vi "FSK_ROBOTIC_ARM_QR_FOUND.vi"() -> ()   [LabVIEW 2025]
uses:
  <vilib>/userDefined/High Color/IMAQdx.ctl
  Program Files/National Instruments/LabVIEW 2025/examples/Instrument IO/Serial/support/Serial - Settings.ctl
  Program Files/National Instruments/LabVIEW 2025/examples/Instrument IO/Serial/support/Serial - XON-XOFF Characters.ctl
  Program Files/National Instruments/LabVIEW 2025/examples/Instrument IO/Serial/support/Serial - ASCII Characters.ctl
  <vilib>/Instr/_visa.llb/VISA Configure Serial Port (Instr).vi
  <vilib>/vision/driver/NI_Vision_Acquisition_Software.lvlib
  <vilib>/vision/NI_Vision_Development_Module.lvlib
panel:
  in  "stop 2":bool
  in  "Termination Character":u8=10 format="%.0x"
  in  "End Write on Termination Character?":bool=TRUE
  in  "VISA resource name":refnum<visa-resource-name>="COM1"
  in  "XON/XOFF Characters":T1={"XON"=enum."DC1", "XOFF"=enum."DC3"}
  in  "Serial Settings":T3={"baud rate"=9600, "data bits"=8, "parity"=enum."None", "stop bits"=10, "flow control"=0} {"flow control" items=["None"=0, "XON/XOFF"=1, "RTS/CTS"=2, "DTR/DSR"=4]; "stop bits" items=["1.0"=10, "1.5"=15, "2.0"=20]; "data bits" min=5 max=8 step=1; "baud rate" items=["75"=75, "110"=110, "134"=134, "150"=150, "300"=300, "600"=600, "1200"=1200, "1800"=1800, "2400"=2400, "4800"=4800, "7200"=7200, "9600"=9600, "14400"=14400, "19200"=19200, "28800"=28800, "38400"=38400, "56000"=56000, "57600"=57600, "115200"=115200, "128000"=128000, "230400"=230400]}
  in  "End Read on Termination Character?":bool=TRUE
  in  "QR a detectar":string(combo)
  out "ROBOTIC ARM":bool
  out "Image":T4(plugin-control)
  in  "stop":bool
  out "ERROR OVERLAY QR":errorcluster
  out "QR FOUND":bool
  out "ERROR QR":errorcluster
  in  "Session In":T5
  out "QR":string
  # "SISTEMA DE CLASIFICACIÓN VISION-DAQ (P1)"
  # "ERRORS"
  # "DATA FOUND"
  # "Deteccíon"
  # "CONFIG"
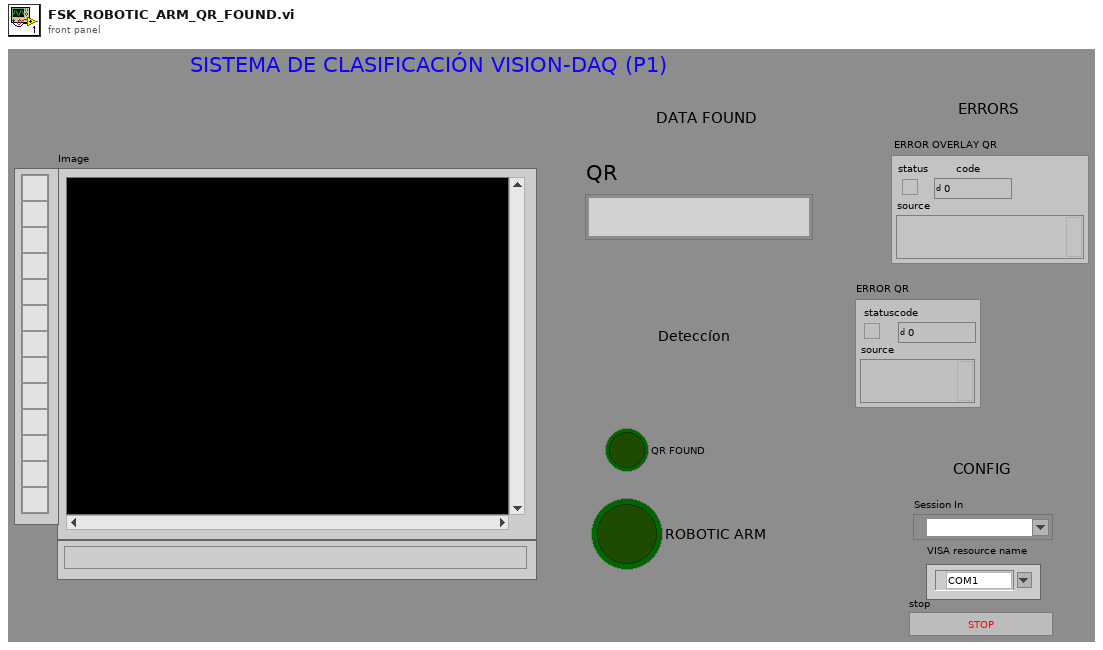
[diagram p1: front panel]
types:
  T1 = typedef "Serial - XON-XOFF Characters.ctl" = cluster{"XON":T2, "XOFF":T2}
  T2 = typedef "Serial - ASCII Characters.ctl" = enum16{"NUL", "SOH", "STX", "ETX", "EOT", "ENQ", "ACK", "BEL", "BS", "HT", "LF", "VT", "FF", "CR", "SO", "SI", "DLE", "DC1", "DC2", "DC3", "DC4", "NAK", "SYN", "ETB", "CAN", "EM", "SUB", "ESC", "FS", "GS", "RS", "US", "SP", "!", "\"", "#", "$", "%", "&", "'", "(", ")", "*", "+", ",", "- (-)", ".", "/", "0", "1", "2", "3", "4", "5", "6", "7", "8", "9", ":", ";", "<", "=", ">", "?", "@", "A", "B", "C", "D", "E", "F", "G", "H", "I", "J", "K", "L", "M", "N", "O", "P", "Q", "R", "S", "T", "U", "V", "W", "X", "Y", "Z", "[", "\\", "]", "^", "_", "`", "a", "b", "c", "d", "e", "f", "g", "h", "i", "j", "k", "l", "m", "n", "o", "p", "q", "r", "s", "t", "u", "v", "w", "x", "y", "z", "{", "|", "}", "~"}
  T3 = typedef "Serial - Settings.ctl" = cluster{"baud rate":u32, "data bits":u16, "parity":enum16{"None", "Odd", "Even", "Mark", "Space"}, "stop bits":u16, "flow control":u16}
  T4 = typedef "IMAQ Image.ctl" = refnum<image>
  T5 = typedef "IMAQdx.ctl" = refnum<k21>
  T6 = typedef "Image Type" = u32
  T7 = typedef "QR Code Report.ctl" = cluster{"Found?":bool, "Data":string, "Bounding Box":cluster{"x":sgl, "y":sgl}[], "Errors Corrected":u32, "Dimensions (Rows/Cols)":u32, "Version":u32, "QR Model":T8, "Stream Mode":T9, "Barcode Polarity":T10, "Mirrored?":bool, "Append Stream Position":u32, "Size of Append Stream":u32, "First EAN-128 ID":i32, "First Alternate Language ID":i32, "Append Stream ID":u32, "Minimum Edge Strength":u32, "Demodulation Mode":T11, "Cell Sample Size":T12, "Cell Filter Mode":T13}
  T8 = typedef "QR Code Model Type.ctl" = i32
  T9 = typedef "QR Code Stream Mode Type.ctl" = i32
  T10 = typedef "Data Matrix Polarity.ctl" = i32
  T11 = typedef "Demodulation Mode.ctl" = i32
  T12 = typedef "Cell Sample Size.ctl" = i32
  T13 = typedef "Cell Filter Mode.ctl" = i32
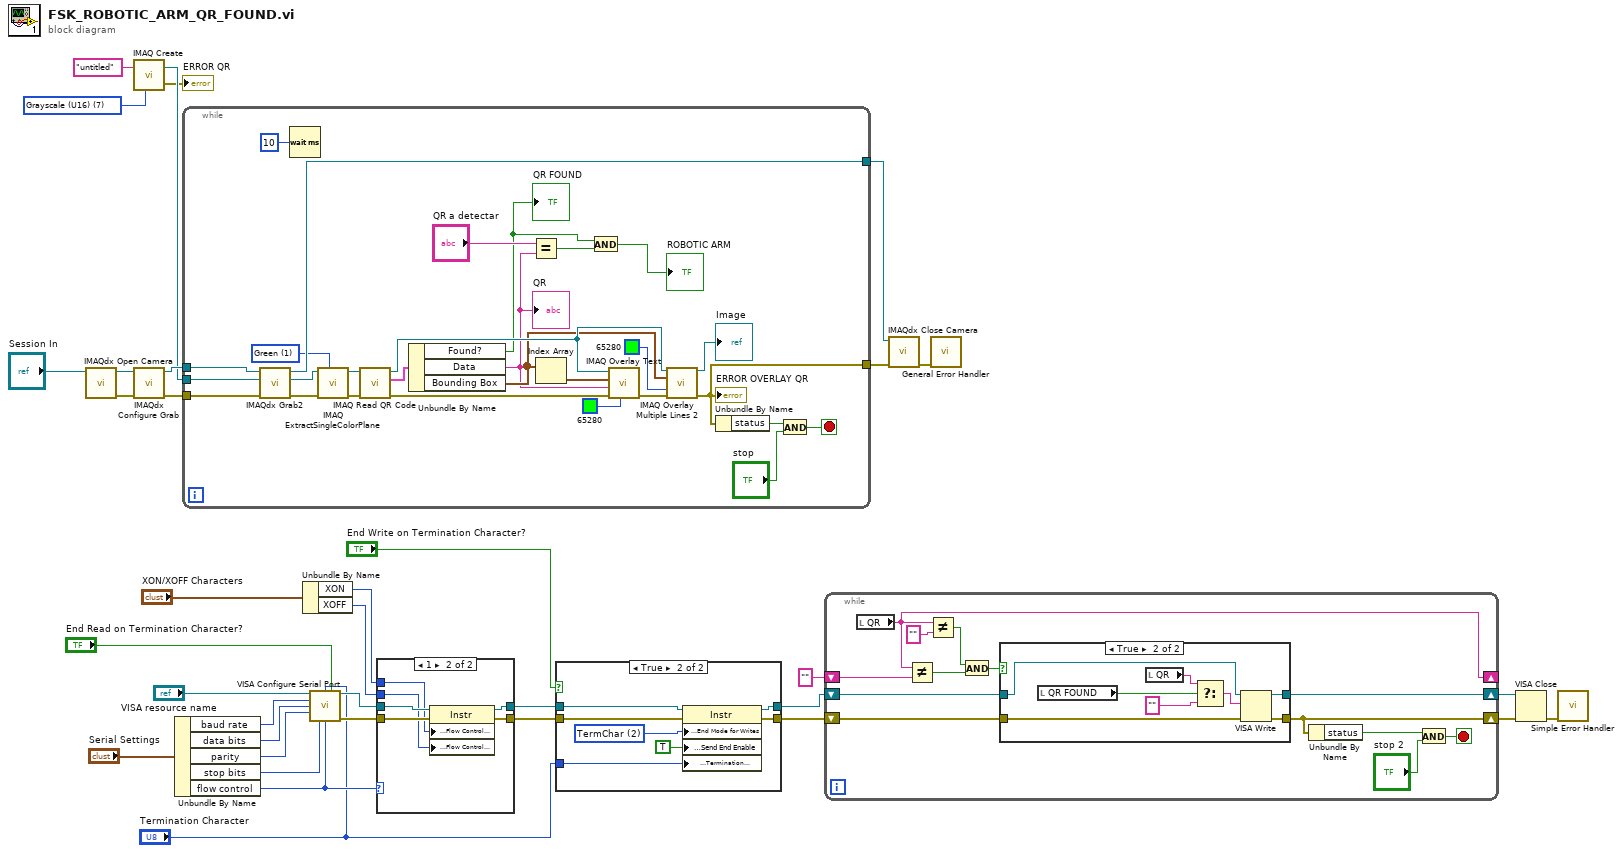
[diagram p0: block diagram]
diagram:
  w29 = T6 7 items=["Grayscale (U8)", "Grayscale (I16)", "Grayscale (SGL)", "Complex (CSG)", "RGB (U32)", "HSL (U32)", "RGB (U64)", "Grayscale (U16)"] ("Image Type")
  n1 = call <vilib>:"IMAQdx Open Camera.vi"("Session In"="Session In") -> ("error out"=w33:errorcluster, "Session Out"=w34:T5)  [unwired: 9 in]
  n2 = call "IMAQ Create"("Image Name"="untitled", "Image Type"=w29) -> ("New Image"=w30:T4, "error out"=→"ERROR QR":errorcluster)  [unwired: 3 in]
  n3 = call <vilib>:"IMAQdx Configure Grab.vi"("error in"=w33, "Session In"=w34) -> ("error out"=w32:errorcluster, "Session Out"=w31:T5)  [unwired: 8 in]
  n4 = Unbundle By Name("Serial Settings") -> ("baud rate"=w16:u32, "data bits"=w17:u16, "parity"=w18:enum16{"None", "Odd", "Even", "Mark", "Space"}, "stop bits"=w19:u16, "flow control"=w12:u16)
  n5 = while {
    tunnel: w32 -> [w63]
    tunnel: w31 -> [w45]
    tunnel: w30 -> [w62]
    tunnel: [w61] -> w27
    tunnel: [w44] -> w25
    stop <- w43 stop-if-true
    w56 = 1 items=["Red", "Green", "Blue", "Hue", "Saturation", "Luminance", "Value", "Intensity"] ("Color Plane")
    n6 = call <vilib>:"IMAQdx Grab2.vi"("error in"=w63, "Image In"=w62, "Session In"=w45) -> ("error out"=w60:errorcluster, "Image Out"=w59:T4, "Session Out"=w61:T5)  [unwired: 5 in, 1 out]
    n7 = Wait (ms)(milliseconds to wait=u32 10) -> ()  [unwired: 1 out]
    n8 = call "IMAQ ExtractSingleColorPlane"("Color Plane"=w56, "error in (no error)"=w60, "Image Src"=w59) -> ("error out"=w58:errorcluster, "Image Dst Out"=w57:T4)  [unwired: 7 in]
    n9 = call "IMAQ Read QR Code"("error in (no error)"=w58, "Image"=w57) -> ("error out"=w49:errorcluster, "QR Code Report"=w55:T7, "Image (duplicate)"=w53:T4)  [unwired: 6 in, 1 out]
    n10 = Unbundle By Name(w55) -> ("Found?"=w38:bool, "Data"=w39:string, "Bounding Box"=w52:cluster{"x":sgl, "y":sgl}[])
    "QR FOUND" <- w38
    "QR" <- w39
    n11 = Equal?(x="QR a detectar", y=w39) -> (x = y?=w37:bool)
    n12 = Index Array(array=w52) -> (element=w48:cluster{"x":sgl, "y":sgl})  [unwired: 1 in]
    n13 = And(x=w38, y=w37) -> (x .and. y?=→"ROBOTIC ARM":bool)
    n14 = call "IMAQ Overlay Text"("Text Color (black)"=u32 65280, "error in (no error)"=w49, "String"=w39, "Origin"=w48, "Image"=w53) -> ("error out"=w50:errorcluster)  [unwired: 5 in, 1 out]
    n15 = call "IMAQ Overlay Multiple Lines 2"("Image"=w53, "Line End Points"=w52, "Color"=u32 65280, "error in (no error)"=w50) -> ("Image Out"=→"Image":T4, "error out"=w44:errorcluster)  [unwired: 10 in]
    "ERROR OVERLAY QR" <- w44
    n16 = Unbundle By Name(w44) -> ("status"=w42:bool)
    n17 = And(x=w42, y="stop") -> (x .and. y?=w43:bool)
  }
  n18 = Unbundle By Name("XON/XOFF Characters") -> ("XON"=w11:T2, "XOFF"=w10:T2)
  n19 = call-poly "VISA Configure Serial Port"("VISA resource name"="VISA resource name", "termination char\n(0xA = '\\n' = LF)"="Termination Character", "Enable Termination\nChar (T)"="End Read on Termination Character?", "baud rate (9600)"=w16, "data bits (8)"=w17, "parity (0:none)"=w18, "stop bits (10: 1 bit)"=w19, "flow control (0:none)"=w12) -> ("VISA resource name out"=w20:refnum<visa-resource-name>, "error out"=w21:errorcluster)  [unwired: 2 in, 4 out]
  n20 = case shown="1" w12 {
    tunnel: [w64 w71] -> w9
    tunnel: [w65 w70] -> w8
    tunnel: w21 -> [w64 w69]
    tunnel: w20 -> [w65 w68]
    tunnel: w11 -> [_ w67]
    tunnel: w10 -> [_ w66]
    frame Default {
    }
    frame 1 {
      n21 = property class="Instr"(reference=w68, error in=w69, "Serial Settings:Flow Control XON Character"=w67, "Serial Settings:Flow Control XOFF Character"=w66) -> (reference out=w70:refnum<visa-resource-name>, error out=w71:errorcluster)
    }
  }
  n22 = case shown="True" "End Write on Termination Character?" {
    tunnel: w8 -> [w72 w80]
    tunnel: w9 -> [w73 w79]
    tunnel: [w72 w74] -> w5
    tunnel: [w73 w78] -> w4
    tunnel: "Termination Character" -> [_ w76]
    frame False {
    }
    frame True {
      w77 = u16 2 items=["None", "LastBit", "TermChar", "Break"] ("Serial Settings:Serial End Mode for Writes")
      n23 = property class="Instr"(reference=w80, error in=w79, "Serial Settings:End Mode for Writes"=w77, "Message Based Settings:Send End Enable"=TRUE, "Message Based Settings:Termination Character"=w76) -> (reference out=w74:refnum<visa-resource-name>, error out=w78:errorcluster)
    }
  }
  n24 = while {
    shift-right: [w91] -> w3
    shift-left: w5 -> [w93]
    shift-right: [w90] -> w2
    shift-left: w4 -> [w92]
    shift-right: [w85] -> _
    shift-left: "" -> [w84]
    stop <- w88 stop-if-true
    n25 = local read "QR"() -> (w85:string)
    n26 = Not Equal?(x=w85, y=w84) -> (x != y?=w82:bool)
    n27 = Not Equal?(x=w85, y="") -> (x != y?=w83:bool)
    n28 = And(x=w83, y=w82) -> (x .and. y?=w81:bool)
    n29 = case shown="True" w81 {
      tunnel: w93 -> [w94 w103]
      tunnel: [w94 w102] -> w91
      tunnel: w92 -> [w95 w101]
      tunnel: [w95 w100] -> w90
      frame False {
      }
      frame True {
        n30 = local read "QR FOUND"() -> (w98:bool)
        n31 = local read "QR"() -> (w99:string)
        n32 = Select(t=w99, s=w98, f="") -> (s? t:f=w96:string)
        n33 = VISA Write(VISA resource name=w103, write buffer=w96, error in (no error)=w101) -> (VISA resource name out=w102:refnum<visa-resource-name>, error out=w100:errorcluster)  [unwired: 1 out]
      }
    }
    n34 = Unbundle By Name(w90) -> ("status"=w89:bool)
    n35 = And(x=w89, y="stop 2") -> (x .and. y?=w88:bool)
  }
  n36 = call <vilib>:"IMAQdx Close Camera.vi"("error in"=w25, "Session In"=w27) -> ("error out"=w24:errorcluster)  [unwired: 9 in]
  n37 = call <vilib>:"General Error Handler.vi"("error in (no error)"=w24) -> ()  [unwired: 10 in, 5 out]
  n38 = VISA Close(VISA resource name=w3, error in (no error)=w2) -> (error out=w13:errorcluster)
  n39 = call <vilib>:"Simple Error Handler.vi"("error in (no error)"=w13) -> ()  [unwired: 1 in, 8 out]
